vi "subCalculate_SwitchROI.vi"(8 "ROI 2 in":T1={"Bin"=4, "ROI"={"x offset"=0, "y offset"=0, "x width"=512, "y width"=512}} {"ROI"."x offset" min=1 max=512 step=1; "ROI"."y offset" min=1 max=512 step=1; "ROI"."x width" min=1 max=512 step=1; "ROI"."y width" min=1 max=512 step=1; "Bin" items=["1x1"=1, "2x2"=2, "4x4"=4]}, 11 "ROI 1 in":T1={"Bin"=4, "ROI"={"x offset"=0, "y offset"=0, "x width"=512, "y width"=512}} {"ROI"."x offset" min=1 max=512 step=1; "ROI"."y offset" min=1 max=512 step=1; "ROI"."x width" min=1 max=512 step=1; "ROI"."y width" min=1 max=512 step=1; "Bin" items=["1x1"=1, "2x2"=2, "4x4"=4]}) -> (0 "ROI 2 out":T1={"Bin"=4, "ROI"={"x offset"=0, "y offset"=0, "x width"=512, "y width"=512}} {"ROI"."x offset" min=1 max=512 step=1; "ROI"."y offset" min=1 max=512 step=1; "ROI"."x width" min=1 max=512 step=1; "ROI"."y width" min=1 max=512 step=1; "Bin" items=["1x1"=1, "2x2"=2, "4x4"=4]}, 3 "ROI 1 out":T1={"Bin"=4, "ROI"={"x offset"=0, "y offset"=0, "x width"=512, "y width"=512}} {"ROI"."x offset" min=1 max=512 step=1; "ROI"."y offset" min=1 max=512 step=1; "ROI"."x width" min=1 max=512 step=1; "ROI"."y width" min=1 max=512 step=1; "Bin" items=["1x1"=1, "2x2"=2, "4x4"=4]})   [LabVIEW 2015]
panel:
  # "Switch  ROI"
  # "ROI 1 out = ROI 2 in\nROI 2 out = ROI 1 in"
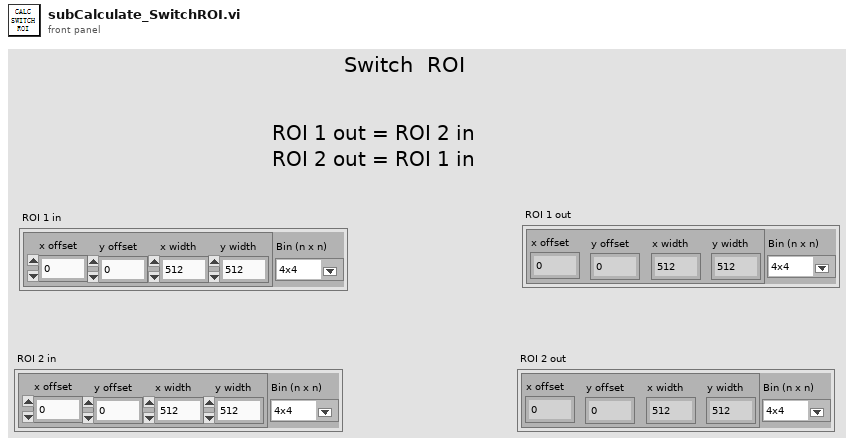
[diagram p1: front panel]
types:
  T1 = cluster{"Bin":u16, "ROI":cluster{"x offset":i32, "y offset":i32, "x width":i32, "y width":i32}}
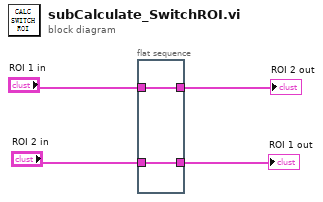
[diagram p0: block diagram]
diagram:
  n1 = flat-sequence {
    tunnel: "ROI 2 in" -> [w6]
    tunnel: [w6] -> w1
    tunnel: "ROI 1 in" -> [w5]
    tunnel: [w5] -> w2
    frame #0 {
    }
  }
  "ROI 1 out" <- w1
  "ROI 2 out" <- w2
